vi "LineCounter.vi"(10 "Mode":T1, 11 "NXT In":T2) -> (2 "NumOfLines":i32, 3 "NXT Out":T2)   [LabVIEW 2012]
uses:
  <vilib>/NXT/Subs/LVHSConnector.ctl
  <vilib>/NXT/LegoClasses/BrickReference/BrickReference.lvclass
  LineCounterControl.ctl
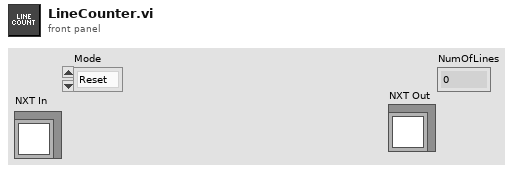
[diagram p1: front panel]
types:
  T1 = typedef "LineCounterControl.ctl" = enum16{"Reset", "Check"}
  T2 = typedef "LVHSConnector.ctl" = refnum<class "BrickReference.lvclass">
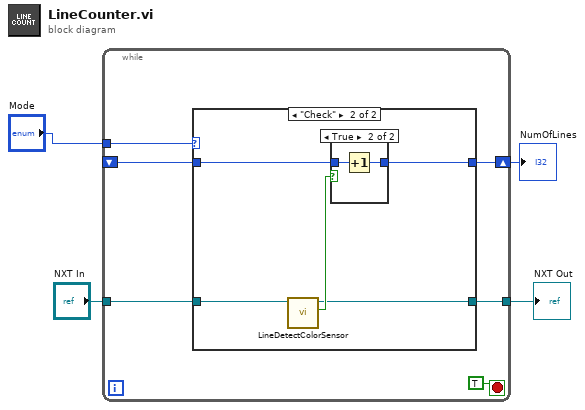
[diagram p0: block diagram]
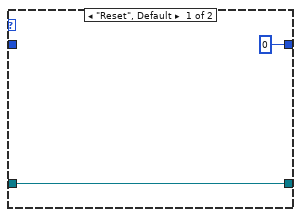
[diagram p2: hidden frame]
diagram:
  n1 = while {
    shift-right: [w9] -> w2
    shift-left: _ -> [w7]
    tunnel: "NXT In" -> [w8]
    tunnel: [w6] -> w3
    tunnel: "Mode" -> [w5]
    stop <- TRUE stop-if-true
    n2 = case shown="\"Check\"" w5 {
      tunnel: [0 ("Numeric") w14] -> w9
      tunnel: w8 -> [w11 w17]
      tunnel: w7 -> [_ w15]
      tunnel: [w11 w13] -> w6
      frame "Reset", Default {
      }
      frame "Check" {
        n3 = call "LineDetectColorSensor.vi"("NXT In"=w17) -> ("CrossedLine?"=w16:bool, "NXT Out"=w13:T2)  [unwired: 9 in]
        n4 = case shown="True" w16 {
          tunnel: w15 -> [w18 w20]
          tunnel: [w18 w19] -> w14
          frame False {
          }
          frame True {
            n5 = Increment(x=w20) -> (x+1=w19:i32)
          }
        }
      }
    }
  }
  "NXT Out" <- w3
  "NumOfLines" <- w2
